vi "XML429_Channel_GetChannelNumber.vi"(0 "Channel in":refnum<k20>, 11 "Error in":errorcluster) -> (4 "Channel out":refnum<k20>, 6 "ChannelNumber":u8, 15 "Error out":errorcluster)   [LabVIEW 2016]
doc: "XML429_Channel_GetChannelNumber"
uses:
  <vilib>/Utility/error.llb/Error Cluster From Error Code.vi
  <vilib>/xml/Close Reference(Node).vi
  <vilib>/xml/Close Reference(NNMap).vi
  <vilib>/ErrorRing/Error Ring.xnode
  <resource>/objmgr/DOMUserDefRef.rc
  <vilib>/xml/NI_XML.lvlib
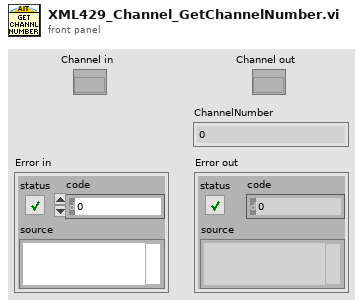
[diagram p1: front panel]
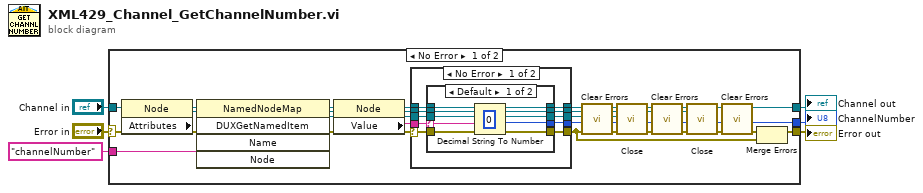
[diagram p0: block diagram]
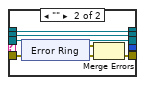
[diagram p2: hidden frame]
diagram:
  n1 = case shown="No Error" "Error in" {
    selector: "Error in" -> [w29 w62]
    tunnel: [w18 w62] -> w5
    tunnel: "Channel in" -> [w28 w61]
    tunnel: [w12 w61] -> w3
    tunnel: [w16 _] -> w2
    tunnel: "channelNumber" ("Name") -> [w7 _]
    frame No Error {
      n2 = property class="Node"(reference=w28, error in=w29) -> (reference out=w13:refnum<k20>, error out=w26:errorcluster, "Attributes"=w27:refnum<k20>)
      n3 = invoke class="NamedNodeMap" method="DUXGetNamedItem"(reference=w27, error in=w26, "Name"=w7) -> (reference out=w11:refnum<k20>, error out=w24:errorcluster, "Node"=w25:refnum<k20>)  [unwired: 2 in, 2 out]
      n4 = property class="Node"(reference=w25, error in=w24) -> (reference out=w9:refnum<k20>, error out=w15:errorcluster, "Value"=w17:string)
      n5 = case shown="No Error" w15 {
        selector: w15 -> [w38 w60]
        tunnel: w17 -> [w36 _]
        tunnel: [w39 _] -> w16
        tunnel: [w37 w60] -> w14
        tunnel: [w34 w59] -> w12
        tunnel: w13 -> [w35 w59]
        tunnel: [w32 w58] -> w10
        tunnel: w11 -> [w33 w58]
        tunnel: [w30 w57] -> w8
        tunnel: w9 -> [w31 w57]
        frame No Error {
          n6 = case shown="Default" w36 {
            selector: w36 -> [w43 _]
            tunnel: [w45 _] -> w39
            tunnel: [w44 w49] -> w37
            tunnel: w38 -> [w44 w48]
            tunnel: [w42 w52] -> w34
            tunnel: w35 -> [w42 w52]
            tunnel: [w41 w51] -> w32
            tunnel: w33 -> [w41 w51]
            tunnel: [w40 w50] -> w30
            tunnel: w31 -> [w40 w50]
            frame Default {
              n7 = Decimal String To Number(string=w43, default (0L)=u8 0 ("default (0 I32)")) -> (number=w45:u8)  [unwired: 1 in, 1 out]
            }
            frame "" {
              n8 = xnode "Error Ring"() -> ("error out"=w47:errorcluster)
              n9 = Merge Errors(w48, w47) -> (w49:errorcluster)
            }
          }
        }
        frame Error {
        }
      }
      n10 = call <vilib>:"Clear Errors.vi"("error in (no error)"=w14) -> ("error out"=w23:errorcluster)  [unwired: 5 in, 1 out]
      n11 = call-poly <vilib>:"Close.vi"("error in (no error)"=w23, "node"=w8) -> ("error out"=w22:errorcluster)  [unwired: 7 in]
      n12 = call <vilib>:"Clear Errors.vi"("error in (no error)"=w22) -> ("error out"=w21:errorcluster)  [unwired: 5 in, 1 out]
      n13 = call-poly <vilib>:"Close.vi"("error in (no error)"=w21, "named node map"=w10) -> ("error out"=w20:errorcluster)  [unwired: 7 in]
      n14 = call <vilib>:"Clear Errors.vi"("error in (no error)"=w20) -> ("error out"=w19:errorcluster)  [unwired: 5 in, 1 out]
      n15 = Merge Errors(w19, w14) -> (w18:errorcluster)
    }
    frame Error {
    }
  }
  "Error out" <- w5
  "Channel out" <- w3
  "ChannelNumber" <- w2
